vi "Lookup Message Size Bytes.vi"(8 "error in (no error)":errorcluster, 10 "Address":u32, 11 "Frames Lookup":variant) -> (0 "error out":errorcluster, 2 "ByteLength":u16)   [LabVIEW 2015, in "Diagnostics Addon Engine.lvlib"]
uses:
  Diagnostics Addon Engine.lvlib
  Shared/Types/Datatable Lookup Positions.ctl
  Shared/Diagnostics Addon Shared.lvlib
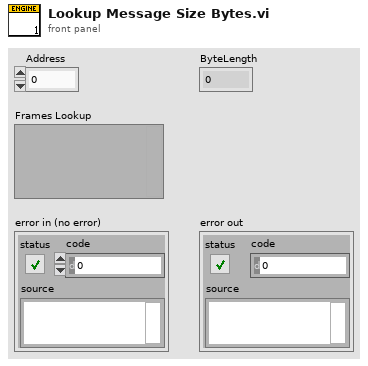
[diagram p1: front panel]
types:
  T1 = typedef "Diagnostics Addon Shared.lvlib/Datatable Lookup Positions.ctl" = cluster{"Offset":i32, "Length":i32, "ByteLength":u16}
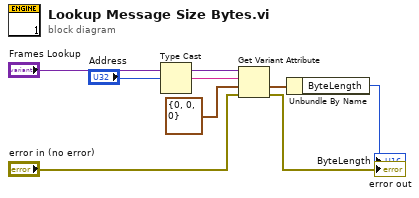
[diagram p0: block diagram]
diagram:
  n1 = Type Cast(x="Address") -> (*(type *) &x=w1:string)  [unwired: 1 in]
  n2 = Get Variant Attribute(Variant="Frames Lookup", name=w1, default value (empty Variant)=T1 {"Offset"=0, "Length"=0, "ByteLength"=0} ("cluster"), error in="error in (no error)") -> (value=w3:T1, error out=→"error out":errorcluster)  [unwired: 2 out]
  n3 = Unbundle By Name(w3) -> ("ByteLength"=→"ByteLength":u16)
